vi "SMBus Block Process Call.vi"(0 "DevType":i32, 1 "CommandCode":u8, 2 "WriteByteCount":u8, 5 "DevIndex":i32, 7 "SMBUSIndex":i32, 9 "SlaveAddr":u8, 11 "error in (no error)":errorcluster, 12 "pWriteData":string, 13 "PEC":u8) -> (4 "pReadData":string, 6 "pReadByteCount":string, 8 "function return":i32, 15 "error out":errorcluster)   [LabVIEW 2012, in "ControlSMBus.lvlib"]
doc: "int WINAPI SMBus_BlockProcessCall(int DevType,int DevIndex,int SMBUSIndex,unsigned char SlaveAddr,unsigned char CommandCode,unsigned char *pWriteData,unsigned char WriteByteCount,unsigned char *pReadData,unsigned char *pReadByteCount,unsigned char PEC);"
uses:
  ControlSMBus.lvlib
  Ginkgo_Driver.dll
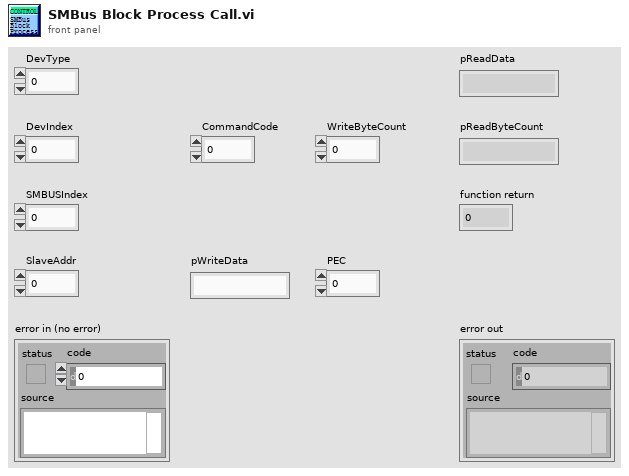
[diagram p1: front panel]
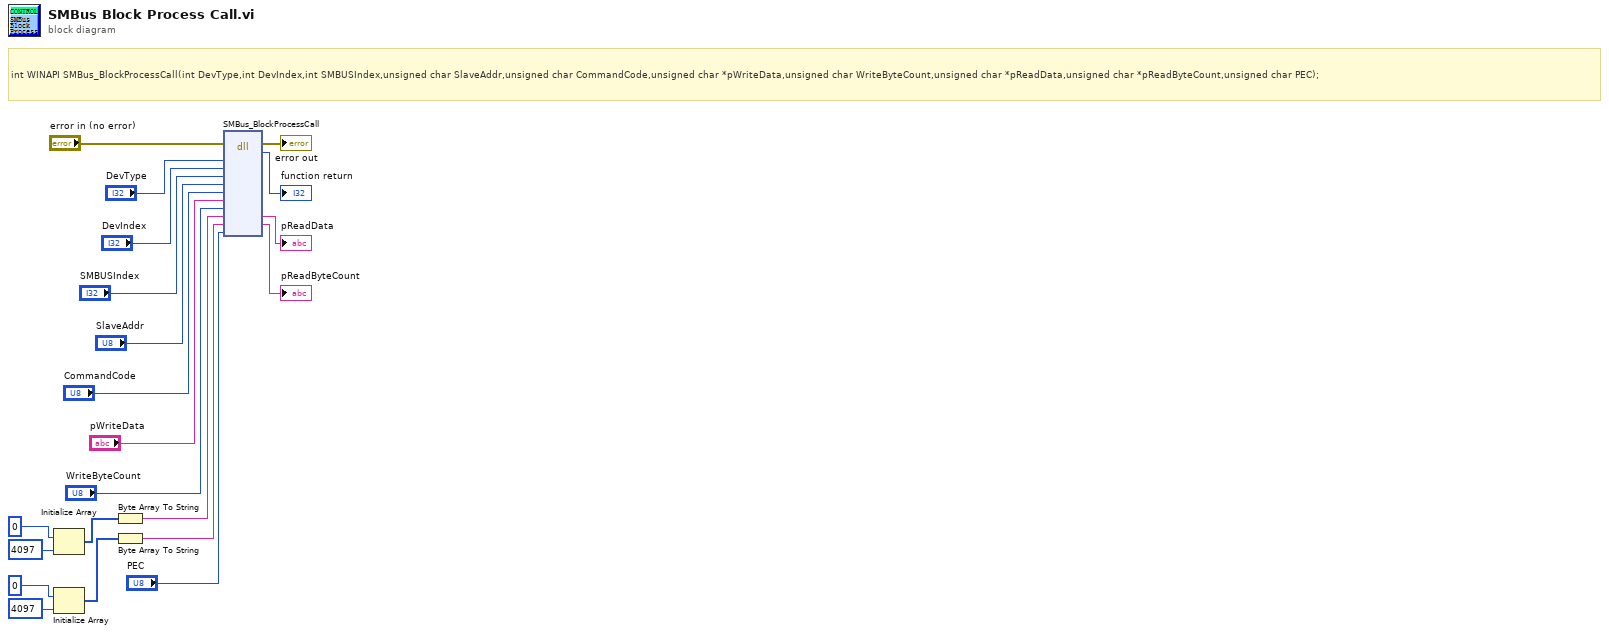
[diagram p0: block diagram]
diagram:
  # "int WINAPI SMBus_BlockProcessCall(int DevType,int DevIndex,int SMBUSIndex,unsigned char SlaveAddr,unsigned char CommandCode,unsigned char *pWriteData,unsigned char WriteByteCount,unsigned char *pReadData,unsigned char *pReadByteCount,unsigned char PEC);"
  n1 = Initialize Array(u8 0 ("element"), 4097 ("dimension size")) -> (w13:u8[])
  n2 = Initialize Array(u8 0 ("element"), 4097 ("dimension size")) -> (w8:u8[])
  n3 = Byte Array To String(unsigned byte array=w13) -> (string=w12:string)
  n4 = Byte Array To String(unsigned byte array=w8) -> (string=w7:string)
  n5 = dll-call lib="E:/Project/vt_ginkgo/truck/Ginkgo Driver/vs2010/Ginkgo_USB-I2C_API_v2.0.3.0/lib/labview_64bit/ControlSMBus/Ginkgo_Driver.*" fn="SMBus_BlockProcessCall"(error in="error in (no error)", "DevType"="DevType", "DevIndex"="DevIndex", "SMBUSIndex"="SMBUSIndex", "SlaveAddr"="SlaveAddr", "CommandCode"="CommandCode", "pWriteData"="pWriteData", "WriteByteCount"="WriteByteCount", "pReadData"=w12, "pReadByteCount"=w7, "PEC"="PEC") -> (error out=→"error out":errorcluster, →"function return":i32, "pReadData"=→"pReadData":string, "pReadByteCount"=→"pReadByteCount":string)  [unwired: 10 in, 1 out]
